vi "Main.vi"() -> ()   [LabVIEW 2019]
uses:
  <vilib>/Platform/TimedLoop/XDataNode/timing_clust.ctl
  <vilib>/Platform/TimedLoop/XDataNode/nitl_modes.ctl
  <vilib>/Platform/TimedLoop/XDataNode/wakeup.ctl
  <vilib>/myRIO/Instrument Drivers/Onboard IO/I2C/typedefs/I2C User Configuration.ctl
  <vilib>/myRIO/Instrument Drivers/Onboard IO/I2C/typedefs/I2C Transfer Rate.ctl
  <vilib>/myRIO/Instrument Drivers/Onboard IO/I2C/typedefs/I2C Reference.ctl
  <vilib>/myRIO/Common/Instrument Driver Framework/Utilities/typedefs/myRIO Generic Hardware Reference.ctl
  <vilib>/myRIO/Common/Instrument Driver Framework/Utilities/typedefs/Hardware Version Enum.ctl
  <vilib>/myRIO/Common/Instrument Driver Framework/Utilities/typedefs/myRIO v1.0 Reference.ctl
  <vilib>/myRIO/Common/Instrument Driver Framework/Utilities/typedefs/Generic FPGA Reference.ctl
  <vilib>/myRIO/Common/Instrument Driver Framework/myRIO v1.0/I2C/typedefs/I2C Channels Enum.ctl
  <vilib>/myRIO/Instrument Drivers/Onboard IO/I2C/typedefs/I2C Configuration.ctl
  <vilib>/userDefined/High Color/nirio_resource_hc.ctl
  <vilib>/myRIO/Common/Instrument Driver Framework/Utilities/vis/Is FPGA Ref Available.vi
  <vilib>/myRIO/Common/Instrument Driver Framework/myRIO v1.0/I2C/vis/myRIO v1.1 Open I2C.vi
  <vilib>/myRIO/Instrument Drivers/Onboard IO/I2C/vis/Configure.vi
  <vilib>/myRIO/Instrument Drivers/Onboard IO/I2C/vis/Write.vi
  <vilib>/myRIO/Common/Instrument Driver Framework/Utilities/vis/Validate Channels.vi
  <vilib>/myRIO/Common/Instrument Driver Framework/myRIO v1.0/I2C/vis/myRIO v1.0 Reserve I2C.vi
  <vilib>/myRIO/Instrument Drivers/Onboard IO/I2C/vis/Write Read.vi
  <vilib>/myRIO/Common/Instrument Driver Framework/myRIO v1.0/UART/vis/myRIO v1.0 Close UART.vi
  <vilib>/myRIO/Common/Instrument Driver Framework/myRIO v1.0/I2C/vis/myRIO v1.0 Build MUX Configuration I2C.vi
  <vilib>/myRIO/Common/Instrument Driver Framework/myRIO v1.0/Resource Manager/vis/myRIO v1.0 Reserve Channel List.vi
  <vilib>/myRIO/Common/Instrument Driver Framework/myRIO v1.0/Resource Manager/vis/myRIO v1.0 Create Configuration List.vi
  <vilib>/myRIO/Common/Instrument Driver Framework/myRIO v1.0/Resource Manager/vis/myRIO v1.0 Reserve Channel.vi
  <vilib>/myRIO/Common/Instrument Driver Framework/myRIO v1.0/Resource Manager/vis/myRIO v1.0 Unreserve Channel.vi
  <vilib>/myRIO/Common/Instrument Driver Framework/myRIO v1.0/Resource Manager/vis/myRIO v1.0 Build Mutex Name.vi
  <vilib>/Utility/VariantDataType/GetNumericInfo.vi
  <vilib>/Utility/error.llb/Error Cluster From Error Code.vi
  <vilib>/myRIO/Common/Instrument Driver Framework/myRIO v1.0/myRIO v1.1 Open.vi
  <vilib>/myRIO/Common/Instrument Driver Framework/Utilities/vis/IO Manager.vi
  <vilib>/myRIO/Common/Instrument Driver Framework/Utilities/vis/Configuration Manager.vi
  <vilib>/myRIO/Common/Instrument Driver Framework/myRIO v1.0/Resource Manager/vis/myRIO v1.0 Configure IO.vi
  <vilib>/myRIO/Common/Instrument Driver Framework/myRIO v1.0/myRIO v1.0 Close.vi
  <vilib>/myRIO/Common/Instrument Driver Framework/myRIO v1.0/I2C/vis/myRIO v1.0 Configure I2C.vi
  <vilib>/myRIO/Common/Instrument Driver Framework/myRIO v1.0/I2C/vis/myRIO v1.0 Write I2C.vi
  <vilib>/myRIO/Instrument Drivers/Onboard IO/I2C/vis/Smart Open.vi
  <vilib>/myRIO/Common/Instrument Driver Framework/myRIO v1.0/I2C/vis/myRIO v1.0 Read I2C.vi
  <vilib>/myRIO/Common/Instrument Driver Framework/Utilities/vis/FPGA Ref Manager.vi
  <vilib>/myRIO/Common/Instrument Driver Framework/myRIO v1.0/myRIO v1.0 Reset FPGA.vi
  <vilib>/myRIO/Common/Instrument Driver Framework/myRIO v1.0/IRQ/vis/myRIO v1.0 IRQ Info FGV.vi
  <vilib>/myRIO/Common/Instrument Driver Framework/myRIO v1.0/IRQ/vis/myRIO v1.0 Timer IRQ Info FGV.vi
  <vilib>/myRIO/Common/Instrument Driver Framework/myRIO v1.0/IRQ/vis/myRIO v1.0 ISR Agent.vi
  <vilib>/myRIO/Instrument Drivers/Utilities/vis/Reset Index.vi
  <vilib>/myRIO/Common/Instrument Driver Framework/myRIO v1.0/Resource Manager/vis/myRIO v1.0 Block Write Resource Manager.vi
  <vilib>/platform/TimedLoop/XDataNode/XDataNode.xnode
  <vilib>/myRIO/Express VI/Onboard IO/I2C/I2C Express VI.xnode
  <vilib>/myRIO/Instrument Drivers/Onboard IO/I2C/vis/myRIO I2C Open.xnode
  <vilib>/myRIO/Instrument Drivers/Utilities/Utilities.lvlib
  <vilib>/Platform/TimedLoop/XDataNode/XDNodeRunTimeDep.lvlib
  <vilib>/myRIO/Instrument Drivers/Onboard IO/I2C/I2C.lvlib
panel:
  out "Magnetic field [G]":cluster{i16, i16, i16}(graph) caption="Waveform Chart"
  out "Z":i16
  out "Y":i16
  out "X":i16
  out "DATA":u8[](array[numeric]) format="%02x"
  in  "[ESC]":bool
  # "DATA_X_H"
  # "DATA_X_L"
  # "DATA_Z_H"
  # "DATA_Z_L"
  # "DATA_Y_H"
  # "DATA_Y_L"
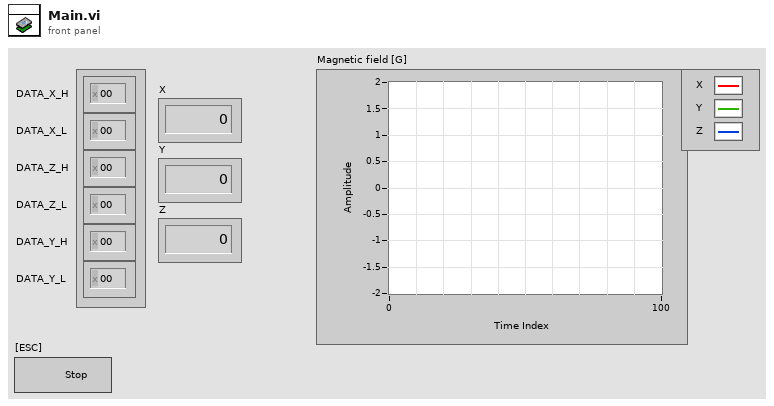
[diagram p1: front panel]
types:
  T1 = typedef "XDNodeRunTimeDep.lvlib/timing_clust.ctl" = cluster{"Expected End [f-1]":u64, "Actual End [f-1]":u64, "Finished Late? [f-1]":bool, "Expected End [i-1]":u64, "Actual End [i-1]":u64, "Finished Late? [i-1]":bool, "Expected Start [i]":u64, "Actual Start [i]":u64, "Expected Start [f]":u64, "Actual Start [f]":u64, "Source Name":string, "Structure Name":string, "Period":i64, "Deadline":i64, "Offset":i64, "Start":i64, "Priority":i32, "Timeout":i32, "Mode":T2, "Wakeup Reason":T3, "Error":errorcluster, "Source Type":string, "Secondary Source Type":string, "Global End Time":u64, "Global Start Time":u64, "Frame Duration":u64, "Iteration Duration":u64, "Assigned CPU":i32, "I/O Scan Engine Mode":u32}
  T2 = typedef "XDNodeRunTimeDep.lvlib/nitl_modes.ctl" = enum32{"No Change", "Process missed periods, maintain original phase", "Discard missed periods, maintain original phase", "Process missed periods, ignore original phase", "Discard missed periods, ignore original phase"}
  T3 = typedef "XDNodeRunTimeDep.lvlib/wakeup.ctl" = enum32{"Normal", "Aborted", "Asynchronous wakeup", "Timing source error", "Timed loop error", "Timeout"}
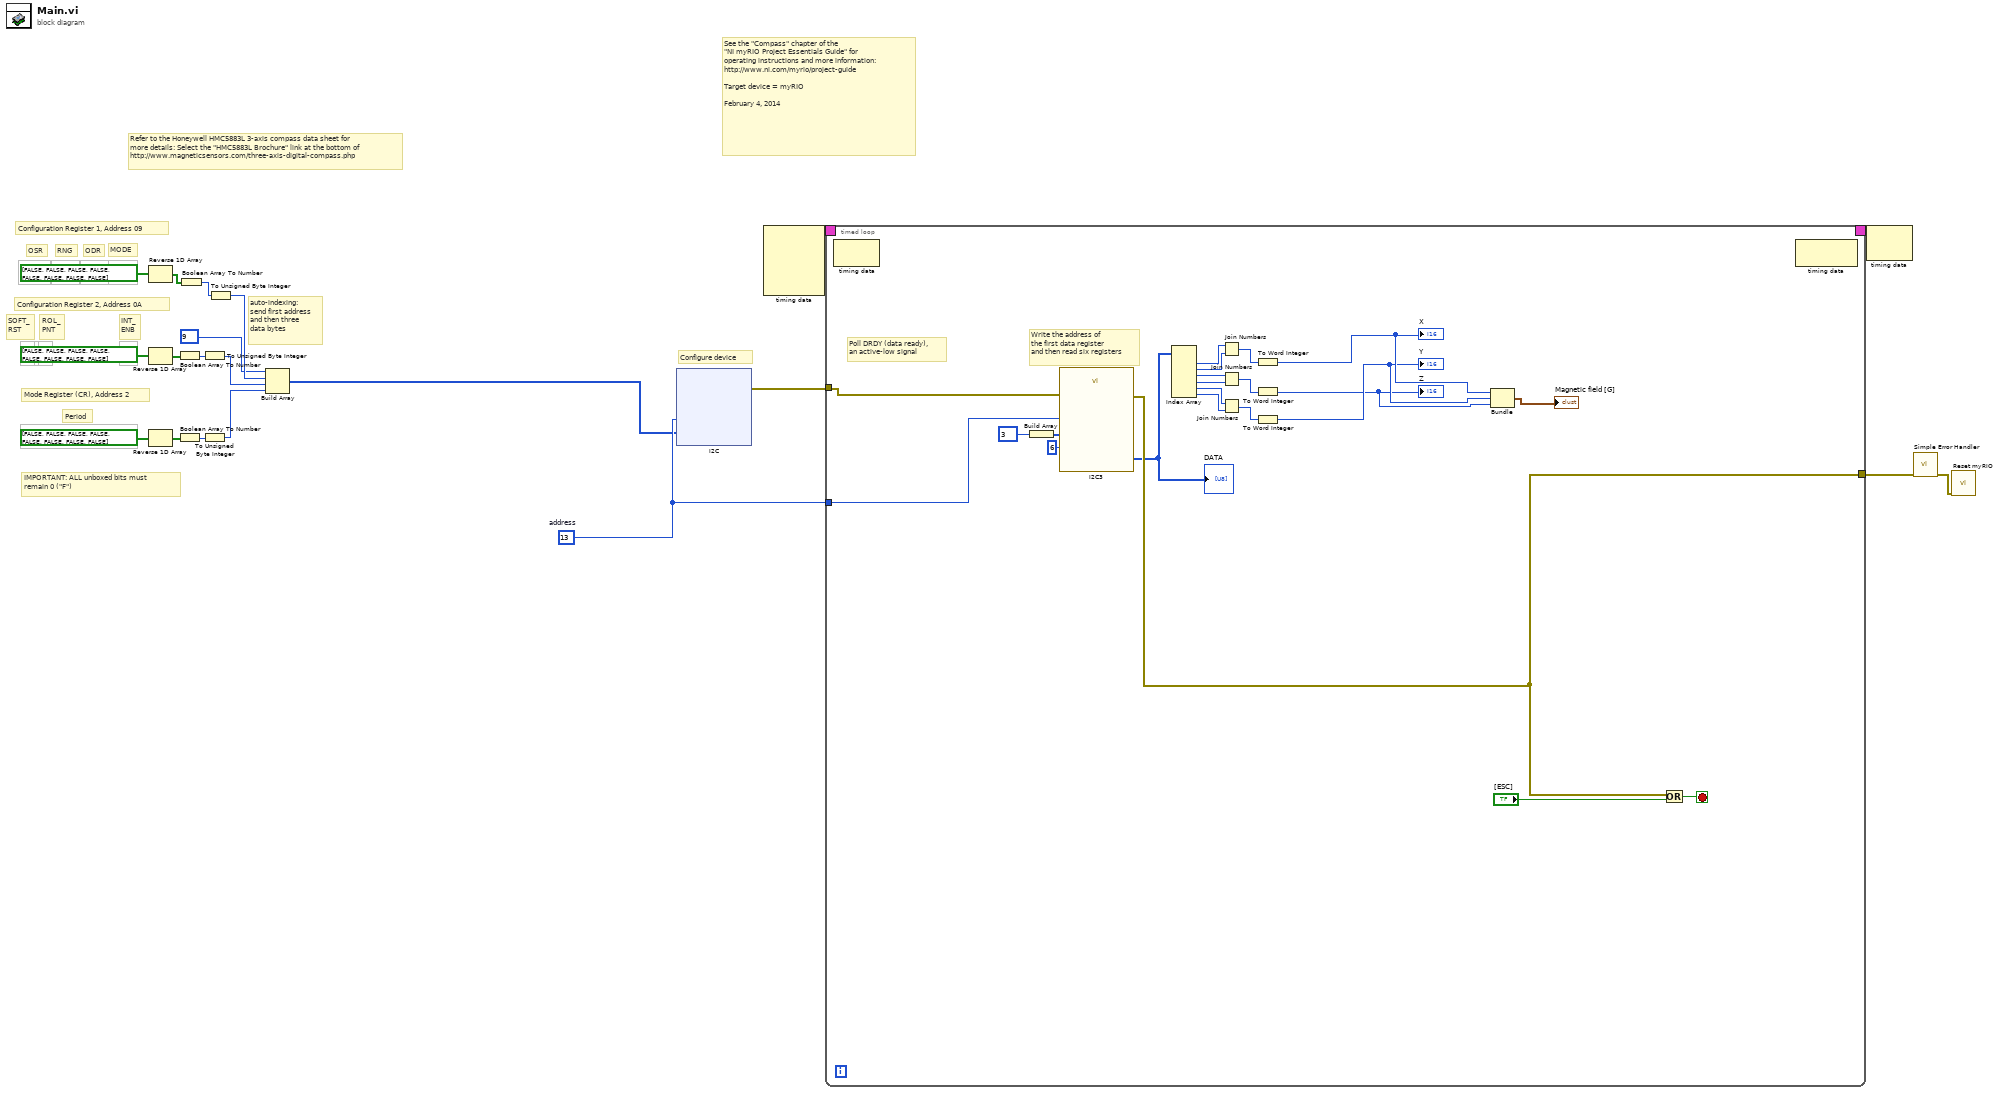
[diagram p0: block diagram]
diagram:
  w17 = u8 13  # address
  # "INT_\nENB"
  # "ROL_\nPNT"
  # "ODR"
  # "auto-indexing:\nsend first address\nand then three\ndata bytes"
  # "IMPORTANT: ALL unboxed bits must\nremain 0 (\"F\")"
  # "Period"
  # "Mode Register (CR), Address 2"
  # "Configuration Register 2, Address 0A"
  # "SOFT_\nRST"
  # "Configuration Register 1, Address 09"
  # "MODE"
  # "RNG"
  # "OSR"
  # "See the \"Compass\" chapter of the\n\"NI myRIO Project Essentials Guide\" for\noperating instructions and more information: \nhttp://www.ni.com/myrio/project-guide\n\nTarget device = myRIO\n\nFebruary 4, 2014"
  # "Refer to the Honeywell HMC5883L 3-axis compass data sheet for \nmore details: Select the \"HMC5883L Brochure\" link at the bottom of\nhttp://www.magneticsensors.com/three-axis-digital-compass.php"
  # "Configure device"
  n1 = Reverse 1D Array(array=bool[] [FALSE, FALSE, FALSE, FALSE, FALSE, FALSE, FALSE, FALSE]) -> (reversed array=w14:bool[])
  n2 = Reverse 1D Array(array=bool[] [FALSE, FALSE, FALSE, FALSE, FALSE, FALSE, FALSE, FALSE]) -> (reversed array=w13:bool[])
  n3 = Reverse 1D Array(array=bool[] [FALSE, FALSE, FALSE, FALSE, FALSE, FALSE, FALSE, FALSE]) -> (reversed array=w12:bool[])
  n4 = Boolean Array To Number(Boolean array=w13) -> (number=w10:u32)
  n5 = Boolean Array To Number(Boolean array=w12) -> (number=w9:u32)
  n6 = Boolean Array To Number(Boolean array=w14) -> (number=w11:u32)
  n7 = To Unsigned Byte Integer(number=w10) -> (unsigned 8bit integer=w7:u8)
  n8 = To Unsigned Byte Integer(number=w9) -> (unsigned 8bit integer=w6:u8)
  n9 = To Unsigned Byte Integer(number=w11) -> (unsigned 8bit integer=w8:u8)
  n10 = Build Array "Build Array"(u8 9 ("address"), w8, w7, w6) -> (w1:u8[])
  n11 = xnode "I2C"("Slave Address (7-bit)"=w17, "Bytes to Write"=w1) -> ("error out"=w18:errorcluster)  [unwired: 1 in]
  n12 = node-c288() -> (w16:T1)  [unwired: 4 in]
  n13 = timed-loop {
    tunnel: [w39] -> w19
    tunnel: w18 -> [w38]
    tunnel: w17 -> [w40]
    timing: w16 -> [_]
    timing-out: [_] -> w15
    stop <- w42 stop-if-true
    # "Write the address of\nthe first data register\nand then read six registers"
    # "Poll DRDY (data ready),\nan active-low signal"
    n14 = node-c288() -> ()  [unwired: 1 in, 1 out]
    n15 = Build Array(u8 3) -> (w25:u8[])
    n16 = call "I2C3"("Slave Address (7-bit)"=w40, "Bytes to Write"=w25, "Byte Count"=u32 6, "error in (no error)"=w38) -> ("Bytes Read"=w28:u8[], "error out"=w39:errorcluster)  [unwired: 22 in]
    "DATA" <- w28
    n17 = Index Array "Index Array"(array=w28) -> (element #1=w37:u8, element #2=w36:u8, element #3=w34:u8, element #4=w33:u8, element #5=w32:u8, element #6=w31:u8)  [unwired: 6 in]
    n18 = Join Numbers(hi=w37, lo=w36) -> ((hi.lo)=w35:u16)
    n19 = Join Numbers(hi=w34, lo=w33) -> ((hi.lo)=w30:u16)
    n20 = Join Numbers(hi=w32, lo=w31) -> ((hi.lo)=w29:u16)
    n21 = To Word Integer(number=w35) -> (16bit integer=w24:i16)
    "X" <- w24
    n22 = To Word Integer(number=w30) -> (16bit integer=w22:i16)
    "Z" <- w22
    n23 = To Word Integer(number=w29) -> (16bit integer=w23:i16)
    "Y" <- w23
    n24 = Bundle(w24, w23, w22) -> (→"Magnetic field [G]":cluster{i16, i16, i16})  [unwired: 1 in]
    n25 = Or(x=w39, y="[ESC]") -> (x .or. y?=w42:bool)
    n26 = node-c288() -> ()  [unwired: 1 in, 1 out]
  }
  n27 = node-c288(w15) -> ()  [unwired: 1 out]
  n28 = call <vilib>:"Simple Error Handler.vi"("error in (no error)"=w19) -> ("error out"=w20:errorcluster)  [unwired: 4 in, 4 out]
  n29 = call <vilib>:"Reset myRIO.vi"("error in (no error)"=w20) -> ()  [unwired: 10 in, 1 out]
